vi "knob.vi"(2 "error in (no error)":errorcluster, 3 "Value":dbl) -> (0 "error out":errorcluster, 1 "Within Limit":bool)   [LabVIEW 2021]
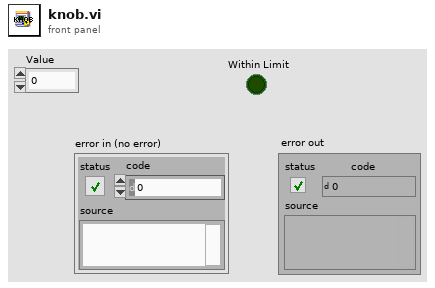
[diagram p1: front panel]
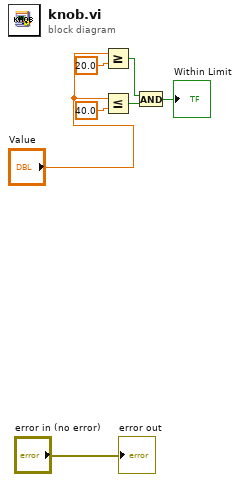
[diagram p0: block diagram]
diagram:
  n1 = Greater Or Equal?(x="Value", y=20.0 ("Lower Limit")) -> (x >= y?=w7:bool)
  n2 = Less Or Equal?(x="Value", y=40.0) -> (x <= y?=w6:bool)
  n3 = And(x=w7, y=w6) -> (x .and. y?=→"Within Limit":bool)
  "error out" <- "error in (no error)"
